vi "Digital Read (SubVI).vi"(3 "error in (no error)":errorcluster, 4 "Digital Input Pin":u8, 5 "Arduino Resource in":T1) -> (0 "error out":errorcluster, 1 "Value":u8, 2 "Arduino Resource out":T1)   [LabVIEW 2015]
uses:
  <vilib>/LabVIEW Interface for Arduino/Type Defs/Arduino Resource.ctl
  <vilib>/LabVIEW Interface for Arduino/Type Defs/Board Type.ctl
  <vilib>/LabVIEW Interface for Arduino/Type Defs/Pin Mode.ctl
  <vilib>/LabVIEW Interface for Arduino/LabVIEW Interface for Arduino.lvlib
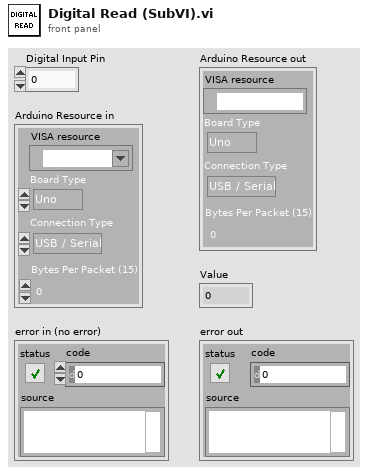
[diagram p1: front panel]
types:
  T1 = typedef "LabVIEW Interface for Arduino.lvlib/Arduino Resource.ctl" = cluster{"VISA resource":refnum<visa-resource-name>, "Board Type":T2, "Connection Type":enum8{"USB / Serial"}, "Bytes Per Packet (15)":u8}
  T2 = typedef "LabVIEW Interface for Arduino.lvlib/Board Type.ctl" = enum16{"Uno", "Dimuelanove w/Atmega 328", "Mega 2560"}
  T3 = typedef "LabVIEW Interface for Arduino.lvlib/Pin Mode.ctl" = enum8{"Input", "Output"}
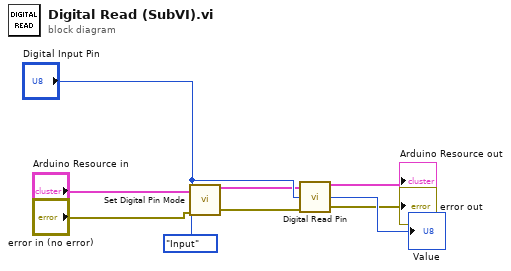
[diagram p0: block diagram]
diagram:
  n1 = call <vilib>:"Set Digital Pin Mode.vi"("Arduino Resource"="Arduino Resource in", "Digital I/O Pin"="Digital Input Pin", "Pin Mode (Input)"=Pin_Mode."Input", "error in"="error in (no error)") -> ("Arduino Resource"=w2:T1, "error out"=w5:errorcluster)  [unwired: 10 in]
  n2 = call <vilib>:"Digital Read Pin.vi"("Arduino Resource"=w2, "Digital I/O Pin (0)"="Digital Input Pin", "error in"=w5) -> ("Arduino Resource"=→"Arduino Resource out":T1, "Value"=→"Value":u8, "error out"=→"error out":errorcluster)  [unwired: 10 in]
